vi "CMD DoSomething.vi"(8 "error in (no error)":errorcluster, 11 "DLP2 in":refnum<class "DLP2.lvclass">) -> (0 "error out":errorcluster, 3 "DLP2 out":refnum<class "DLP2.lvclass">)   [LabVIEW 2022 SP3, in "DLP2.lvclass"]
doc: "Developed by Kevin Thompson\nkevin@thompsonengineering.net\n\nCopyright 2018\nThompson Engineering, LLC"
uses:
  DLP2.lvclass
  DLP2.lvclass/DLP2.ctl
  DataTypes/AsynCmd_Temp01--enum.ctl
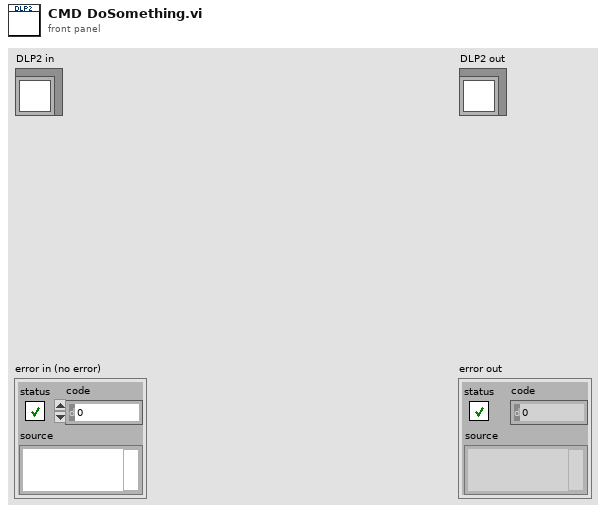
[diagram p1: front panel]
types:
  T1 = typedef "DLP2.lvclass/AsynCmd_Temp01--enum.ctl" = enum16{"LoadTiffImage"}
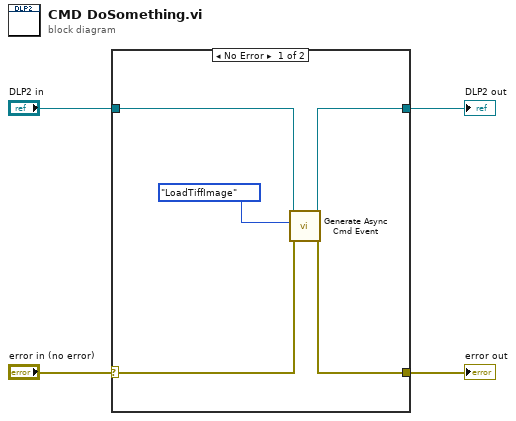
[diagram p0: block diagram]
diagram:
  n1 = case shown="No Error" "error in (no error)" {
    selector: "error in (no error)" -> [w7 w11]
    tunnel: [w6 w11] -> w3
    tunnel: [w8 w10] -> w1
    tunnel: "DLP2 in" -> [w9 w10]
    frame No Error {
      n2 = call "Generate Async Cmd Event.vi"("error in (no error)"=w7, "AsyncCmd"=AsynCmd_Temp01--enum."LoadTiffImage", "DLP2 in"=w9) -> ("error out"=w6:errorcluster, "DLP2 out"=w8:refnum<class "DLP2.lvclass">)  [unwired: 7 in]
    }
    frame Error {
    }
  }
  "error out" <- w3
  "DLP2 out" <- w1
